vi "Watch_Directory3.vi"() -> ()   [LabVIEW 2015]
uses:
  <vilib>/Utility/config.llb/Read Key (String).vi
  <userlib>/caLab/Private/Get_PV-1D.vi
  <vilib>/Utility/config.llb/NI_LVConfig.lvlib
panel:
  out "Numeric":i32
  out "path":path
  out "concatenated string 8":string
  out "LOGBOOK":string
  out "PATH HSnapjpeg":string
  out "PATH SESdata":string
  out "PV name array":string[](array[string])
  out "BL132:CONFIG":path=path "S:/INI/BL132.INI"
  out "ELOGD_SERVER":string
  out "concatenated string 7":string
  in  "error out 2":errorcluster
  out "error out":errorcluster
  out "EPICS_PVs":string
  out "subarray 2":dbl[](array[numeric])
  out "subarray":dbl[](array[numeric])
  out "concatenated string 3":string
  out "standard error 5":string
  out "standard output 5":string
  out "SEStxt Previous":string
  out "SEStxt":bool
  out "standard output 4":string
  out "standard error 4":string
  out "concatenated string 2":string
  in  "SES_Filter txt":string="*.txt"
  out "SEStxt Current":string
  out "concatenated string 6":string
  out "standard error 3":string
  out "standard output 3":string
  in  "Submit":bool
  in  "HSnap_Filter jpg":string="*.jpg"
  in  "ELOG:HSnap_Maindir":string="S:\\HyperSnap\\"
  out "HSnap Current":string
  out "concatenated string 5":string
  in  "ELOGHSnap_Subdir":string
  out "HSnap Previous":string
  out "HyperSnap":bool
  out "standard output 2":string
  out "standard error 2":string
  out "concatenated string 4":string
  in  "ELOG:SES_maindir":string="P:\\b_ogasawara\\bl13-0\\bl13-2\\dt_SES100\\"
  in  "stop 2":bool
  in  "ELOG_MESSAGE":string caption="Message to ELOG  BL132:Message"
  out "SESpath":path
  in  "ELOG:SES_subdir":string="2017\\BL132\\"
  out "PV Names (dup)":string[](array[string])
  out "concatenated string":string
  out "standard error":string
  out "standard output":string
  out "SESibw":bool
  out "SESibw Previous":string
  in  "SES_Filter ibw":string="*.ibw"
  out "SESibw Current":string
  # "Set a folder to watch using the\nPath control. You can also\nset a filter for a certain type\nof file to watch for (such as\n*.bmp). Then run the\nexample. Whenever you create\na new file in that directory that\nmatches the filter, New File Name\nwill update to let you know the\nnew file name."
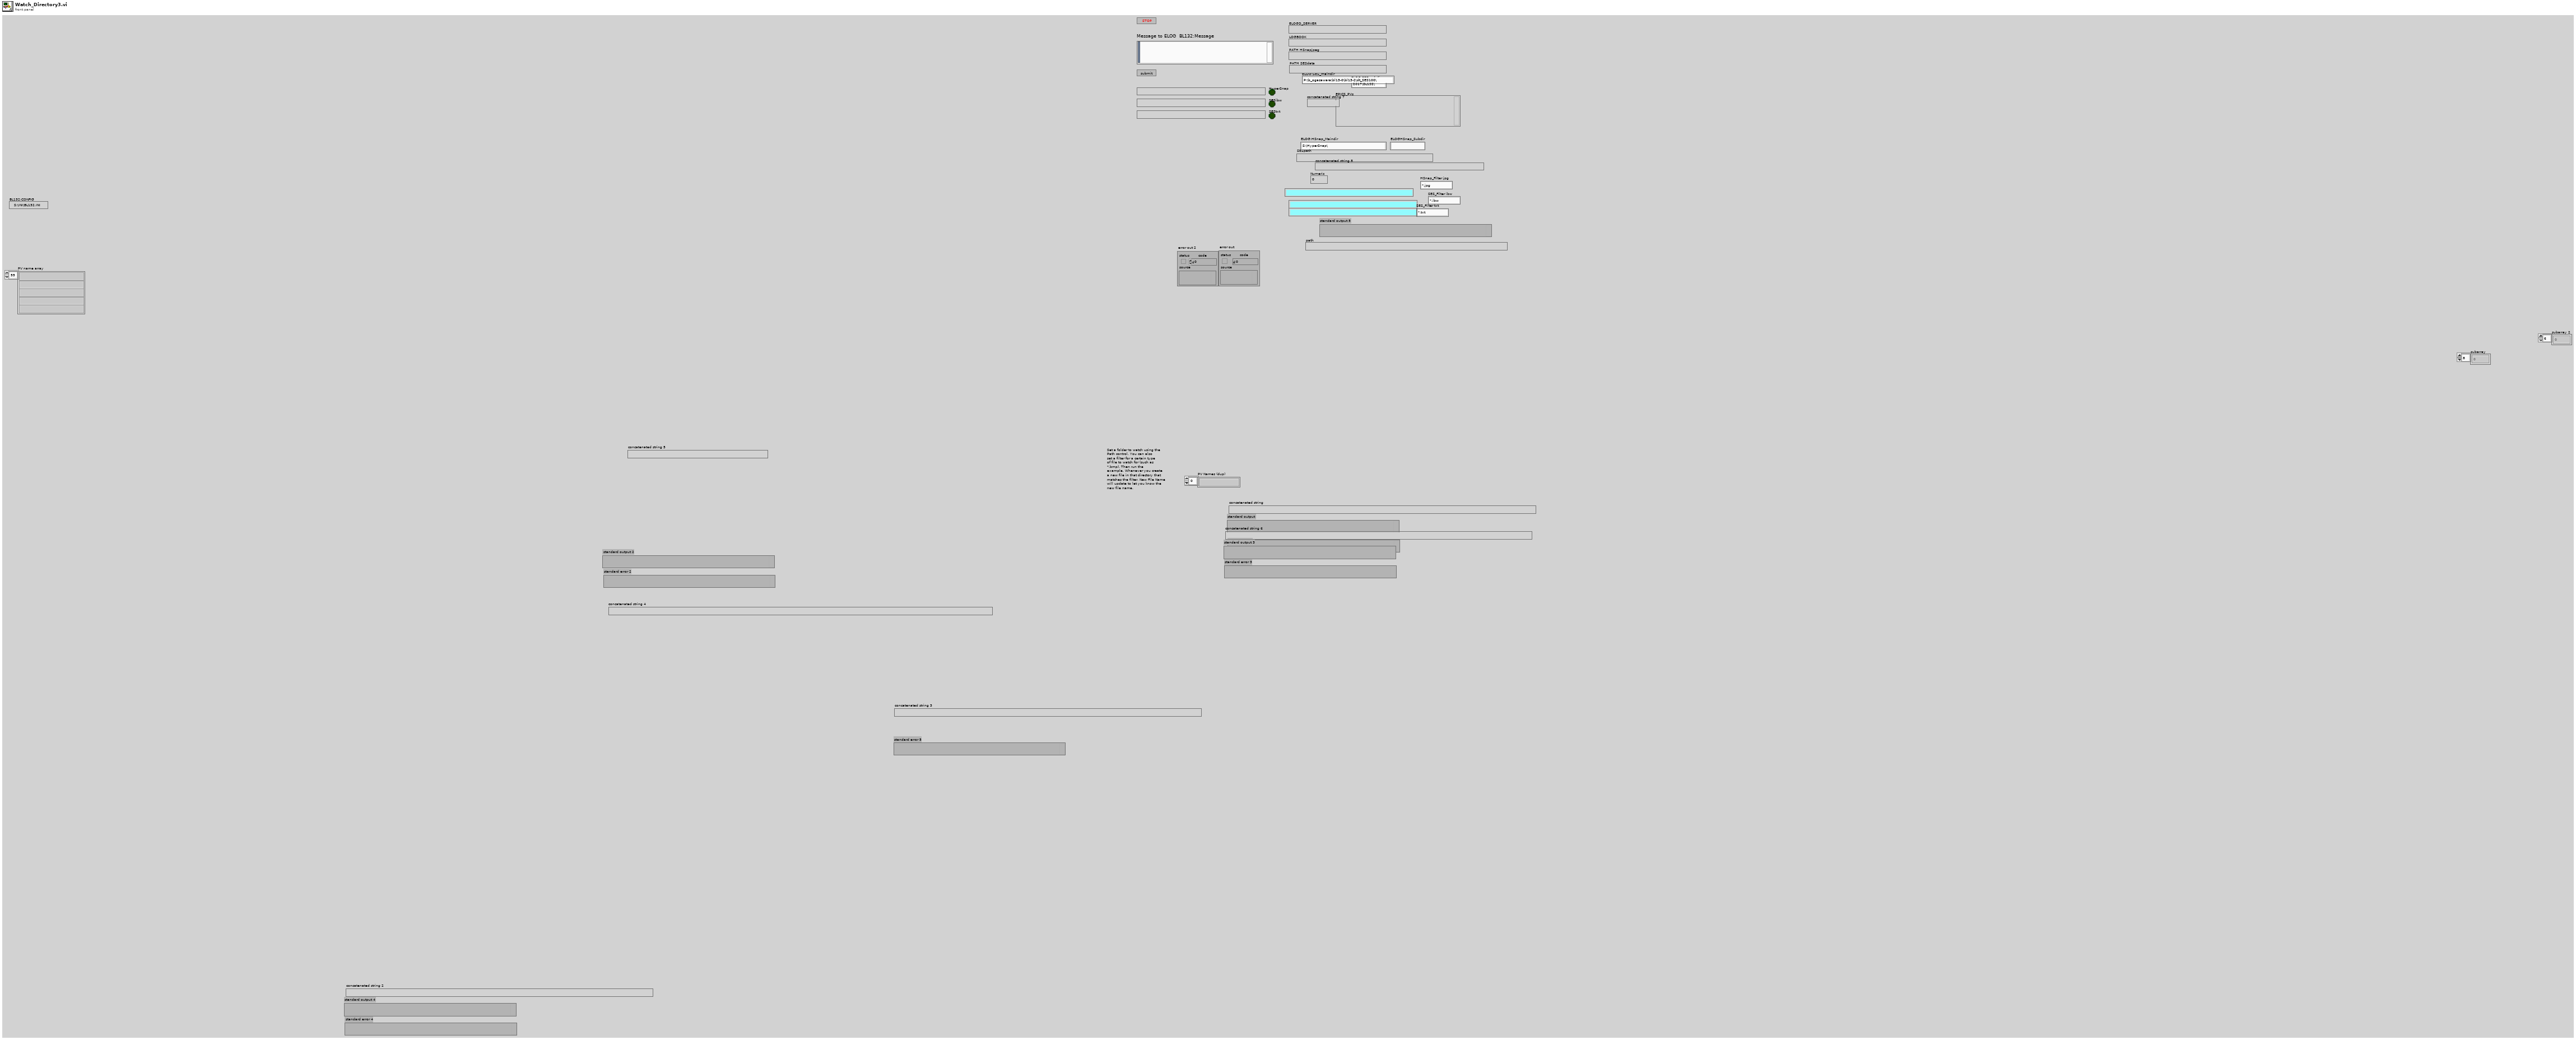
[diagram p1: front panel]
types:
  T1 = typedef "NI_LVConfig.lvlib/Config Data RefNum.ctl" = refnum<k1>
  T2 = enum16{"open", "replace", "create", "open or create", "replace or create", "replace or create with confirmation"}
  T3 = typedef "imagedata.ctl" = cluster{"image type":i32, "image depth":i32, "image":u8[], "mask":u8[], "colors":u32[], "Rectangle":cluster{"left":i16, "top":i16, "right":i16, "bottom":i16}}
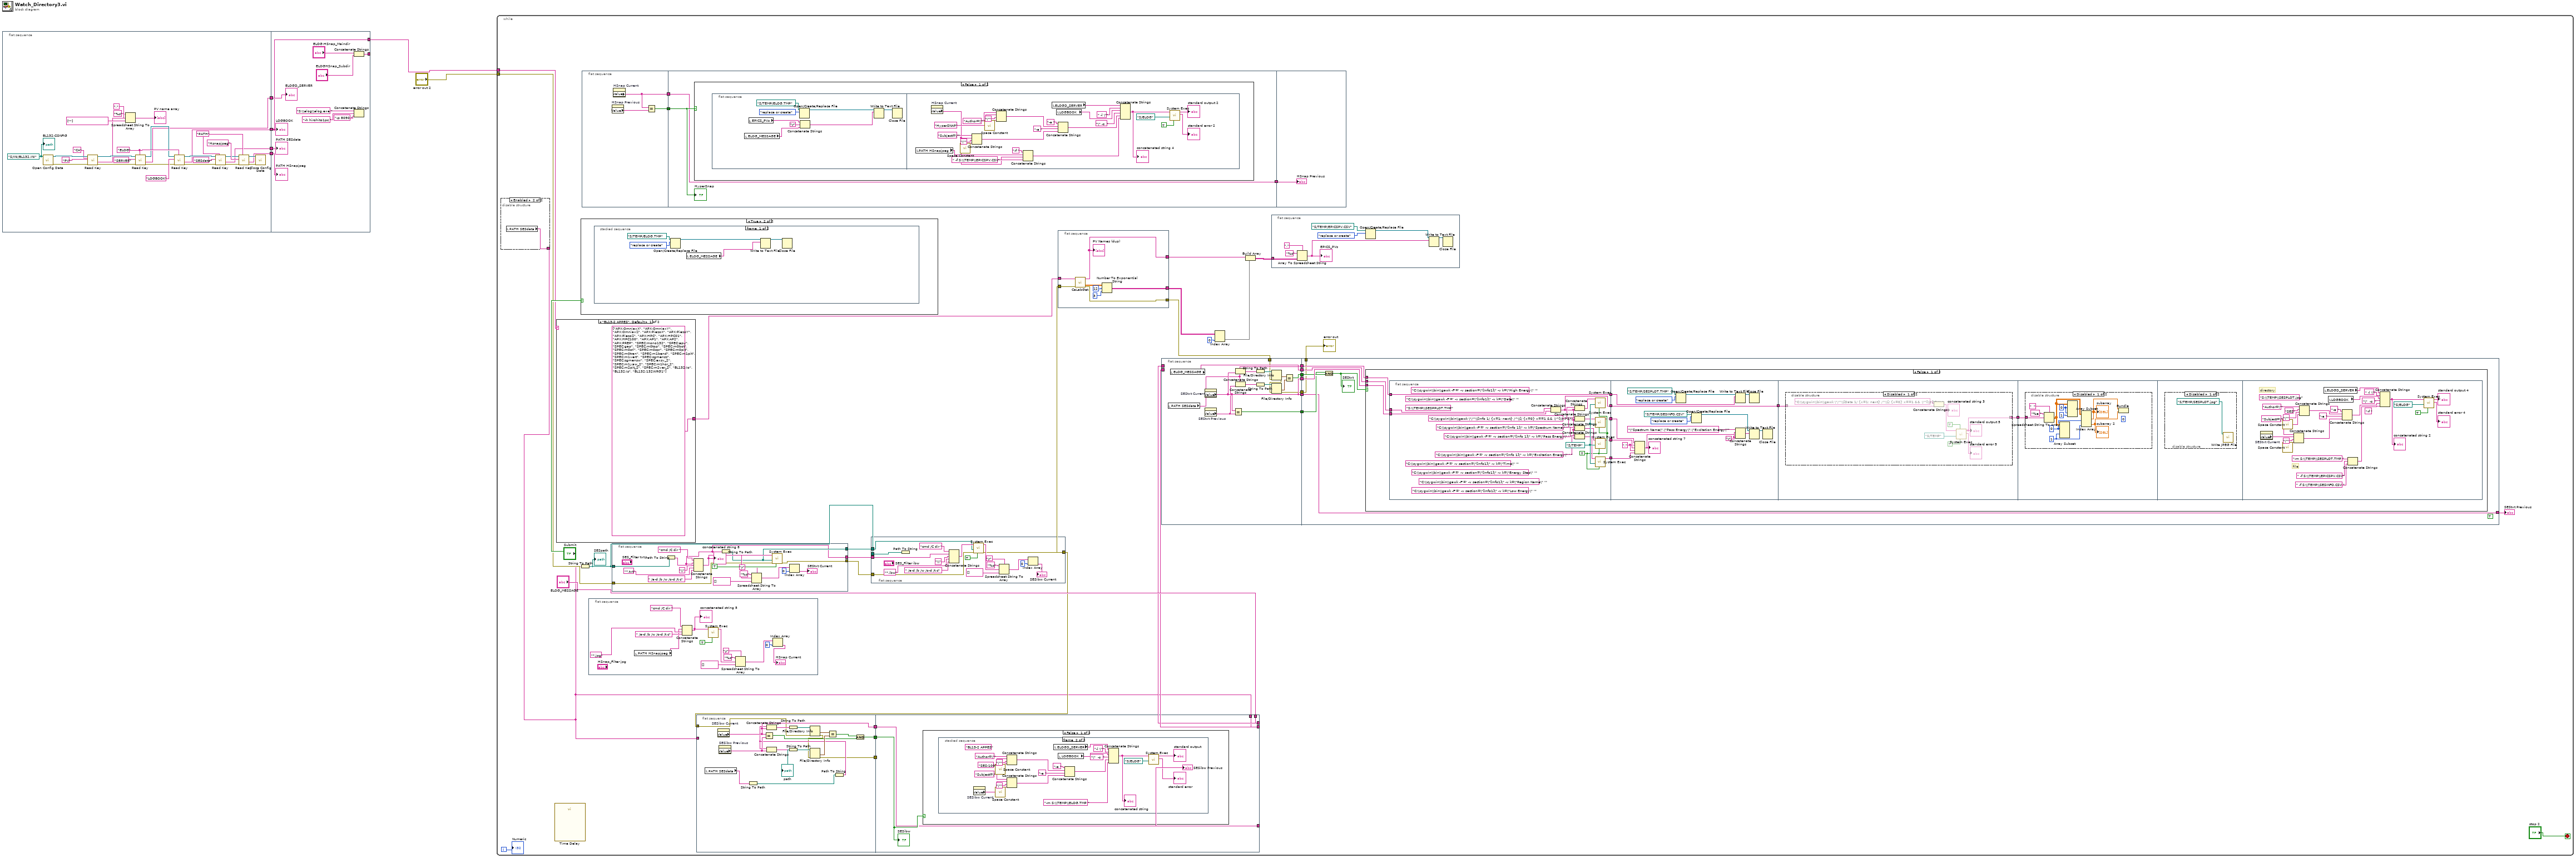
[diagram p0: block diagram]
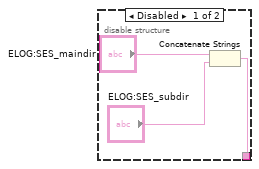
[diagram p2: hidden frame]
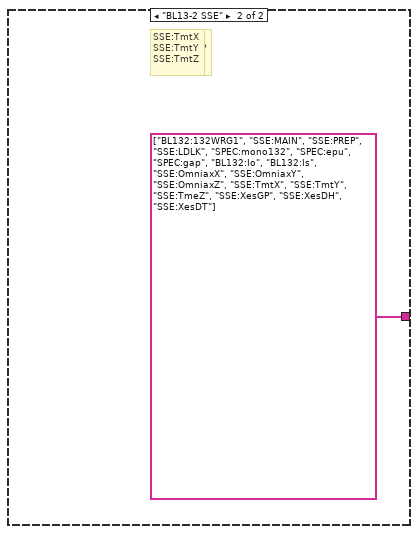
[diagram p3: hidden frame]
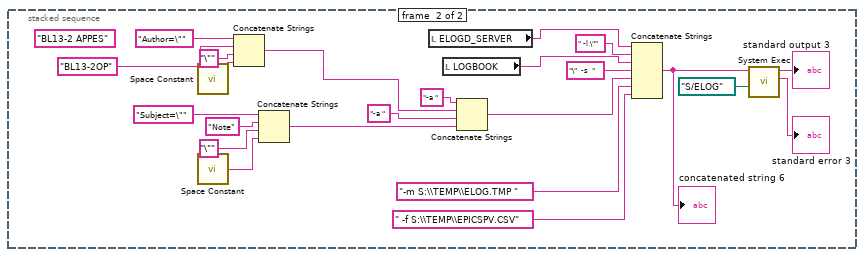
[diagram p9: hidden frame]
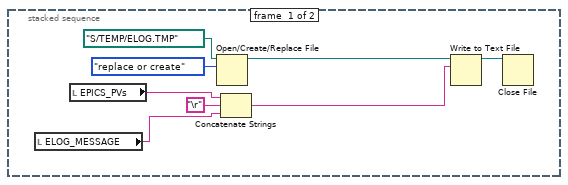
[diagram p11: hidden frame]
diagram:
  n1 = flat-sequence {
    tunnel: [w11] -> w4
    tunnel: [w10] -> w3
    tunnel: [w9] -> w2
    tunnel: [w8] -> w1
    tunnel: [w37] -> w5
    tunnel: [w43] -> _
    tunnel: w4 -> [w40]
    tunnel: w3 -> [w39]
    tunnel: w2 -> [w38]
    tunnel: w1 -> [w37]
    frame #0 {
      w12 = "PATH" ("section")
      w36 = path "S:/INI/BL132.INI" ("configuration file path")
      w18 = "ELOG" ("key")
      n2 = call <vilib>:"Open Config Data.vi"("configuration file path"=w36) -> ("error out"=w25:errorcluster, "refnum"=w33:T1)  [unwired: 8 in, 1 out]
      n3 = call-poly <vilib>:"Read Key.vi"("section"="CA", "error in (no error)"=w25, "key"="PV", "refnum"=w33) -> ("error out"=w26:errorcluster, "value"=w27:string, "refnum out"=w30:T1)  [unwired: 4 in, 1 out]
      n4 = Spreadsheet String To Array(delimiter (Tab)=",", format string="%s", spreadsheet string=w27, array type (2D Dbl)=string[] [""] ("Strings []")) -> (array=→"PV name array":string[])
      n5 = call-poly <vilib>:"Read Key.vi"("section"=w18, "error in (no error)"=w26, "key"="SERVER" ("section"), "refnum"=w30) -> ("error out"=w14:errorcluster, "value"=w9:string, "refnum out"=w16:T1)  [unwired: 4 in, 1 out]
      n6 = call-poly <vilib>:"Read Key.vi"("section"=w18, "error in (no error)"=w14, "key"="LOGBOOK", "refnum"=w16) -> ("error out"=w13:errorcluster, "value"=w8:string, "refnum out"=w15:T1)  [unwired: 4 in, 1 out]
      n7 = call-poly <vilib>:"Read Key.vi"("section"=w12, "error in (no error)"=w13, "key"="SESdata", "refnum"=w15) -> ("error out"=w20:errorcluster, "value"=w11:string, "refnum out"=w22:T1)  [unwired: 4 in, 1 out]
      n8 = call-poly <vilib>:"Read Key.vi"("section"=w12, "error in (no error)"=w20, "key"="Hsnapjpeg", "refnum"=w22) -> ("error out"=w19:errorcluster, "value"=w10:string, "refnum out"=w21:T1)  [unwired: 4 in, 1 out]
      n9 = call <vilib>:"Close Config Data.vi"("error in (no error)"=w19, "refnum"=w21) -> ()  [unwired: 8 in, 2 out]
      "BL132:CONFIG" <- w36
    }
    frame #1 {
      n10 = Concatenate Strings("ELOG:HSnap_Maindir", "ELOGHSnap_Subdir") -> (w43:string)
      n11 = Concatenate Strings("S:\\elog\\elog.exe " ("command line"), "-h hirohito1pc " ("command line"), "-p 8090 " ("string")) -> ()  [unwired: 1 out]
      "ELOGD_SERVER" <- w38
      "PATH SESdata" <- w40
      "PATH HSnapjpeg" <- w39
      "LOGBOOK" <- w37
    }
  }
  n12 = while {
    tunnel: "error out 2" -> [w59]
    tunnel: w5 -> [w56]
    i -> [w47]
    stop <- "stop 2" stop-if-true
    n13 = disable-structure shown="Enabled" {
      disable-tunnel: [w84 w87] -> w48
      frame Disabled {
        n14 = Concatenate Strings("ELOG:SES_maindir", "ELOG:SES_subdir") -> (w84:string)
      }
      frame Enabled {
        n15 = local read "PATH SESdata"() -> (w87:string)
      }
    }
    n16 = call "Time Delay"() -> ()  [unwired: 11 in, 1 out]
    n17 = case shown="\"BL13-2 APPES\", Default" w56 {
      tunnel: [string[] ["APX:OmniaxX", "APX:OmniaxY", "APX:OmniaxZ", "APX:PiezoX", "APX:PiezoY", "APX:PiezoZ", "APX:HPC", "APX:HPC01", "APX:HPC100", "APX:AP1", "APX:AP2", "APX:PREP", "SPEC:mono132", "SPEC:epu", "SPEC:gap", "SPEC:m0top", "SPEC:m0bot", "SPEC:m0srl", "SPEC:m0spr", "SPEC:m0pit", "SPEC:m0tran", "SPEC:m1bend", "SPEC:m1pit", "SPEC:m1vert", "SPEC:sgmensz", "SPEC:sgmensw", "SPEC:exsv_2", "SPEC:m1yaw_2", "SPEC:m1hor_2", "SPEC:m2pit_2", "SPEC:m2ver_2", "BL132:Io", "BL132:Is", "BL132:132WRG1"] string[] ["BL132:132WRG1", "SSE:MAIN", "SSE:PREP", "SSE:LDLK", "SPEC:mono132", "SPEC:epu", "SPEC:gap", "BL132:Io", "BL132:Is", "SSE:OmniaxX", "SSE:OmniaxY", "SSE:OmniaxZ", "SSE:TmtX", "SSE:TmtY", "SSE:TmeZ", "SSE:XesGP", "SSE:XesDH", "SSE:XesDT"]] -> w62
      frame "BL13-2 APPES", Default {
      }
      frame "BL13-2 SSE" {
        # "SSE:TmtX\nSSE:TmtY\nSSE:TmtZ"
        # "SSE:XesDT\nSSE:Xes:GP\nSSE:XesDT"
      }
    }
    n18 = String To Path(string=w48) -> (path=w73:path)
    "SESpath" <- w73
    n19 = case shown="True" "Submit" {
      frame False {
      }
      frame True {
        n20 = stacked-sequence {
          frame #0 {
            n21 = Open/Create/Replace File(file path (use dialog)=path "S:/TEMP/ELOG.TMP", operation (0:open)=T2."replace or create") -> (refnum out=w246:refnum<file>)  [unwired: 4 in, 2 out]
            n22 = local read "ELOG_MESSAGE"() -> (w242:string)
            n23 = Write to Text File(file (use dialog)=w246, text=w242) -> (refnum out=w245:refnum<file>)  [unwired: 2 in, 2 out]
            n24 = Close File(refnum=w245) -> ()  [unwired: 1 in, 2 out]
          }
          frame #1 {
            (unwired) "BL13-2 APPES"
            n25 = call <vilib>:"Space Constant.vi"() -> ("String"=w257:string)
            n26 = call <vilib>:"Space Constant.vi"() -> ("String"=w258:string)
            n27 = Concatenate Strings("Author=\"" ("string"), "BL13-2OP", "\"" ("string"), w257) -> (w255:string)
            n28 = Concatenate Strings("Subject=\"" ("string"), "Note" ("string"), "\"" ("string"), w258) -> (w253:string)
            n29 = local read "ELOGD_SERVER"() -> (w248:string)
            n30 = local read "LOGBOOK"() -> (w247:string)
            n31 = Concatenate Strings("-a ", w255, "-a " ("string"), w253) -> (w254:string)
            n32 = Concatenate Strings(w248, " -l \"" ("command line"), w247, "\"  -s  " ("command line"), w254, "-m S:\\TEMP\\ELOG.TMP " ("string"), " -f S:\\TEMP\\EPICSPV.CSV" ("string")) -> (w266:string)
            "concatenated string 6" <- w266
            n33 = call <vilib>:"System Exec.vi"("working directory"=path "S:/ELOG", "command line"=w266) -> ("standard error"=→"standard error 3":string, "standard output"=→"standard output 3":string)  [unwired: 6 in, 2 out]
          }
        }
      }
    }
    n34 = flat-sequence {
      tunnel: [w283] -> w81
      tunnel: [w284] -> w80
      tunnel: w81 -> [w286]
      tunnel: [w286] -> w79
      tunnel: w80 -> [w287]
      tunnel: w79 -> [w322]
      frame #0 {
        n35 = property on="HSnap Previous" class="Str"() -> ("Value"=w285:string)  [unwired: 2 in, 2 out]
        n36 = property on="HSnap Current" class="Str"() -> ("Value"=w283:string)  [unwired: 2 in, 2 out]
        n37 = Equal?(x=w283, y=w285) -> (x = y?=w284:bool)
      }
      frame #1 {
        n38 = case shown="False" w287 {
          frame False {
            n39 = flat-sequence {
              frame #0 {
                n40 = local read "ELOG_MESSAGE"() -> (w288:string)
                n41 = local read "EPICS_PVs"() -> (w289:string)
                n42 = Open/Create/Replace File(file path (use dialog)=path "S:/TEMP/ELOG.TMP", operation (0:open)=T2."replace or create") -> (refnum out=w295:refnum<file>)  [unwired: 4 in, 2 out]
                n43 = Concatenate Strings(w289, "\r", w288) -> (w290:string)
                n44 = Write to Text File(file (use dialog)=w295, text=w290) -> (refnum out=w294:refnum<file>)  [unwired: 2 in, 2 out]
                n45 = Close File(refnum=w294) -> ()  [unwired: 1 in, 2 out]
              }
              frame #1 {
                n46 = local read "PATH HSnapjpeg"() -> (w297:string)
                n47 = property on="HSnap Current" class="Str"() -> ("Value"=w296:string)  [unwired: 2 in, 2 out]
                n48 = call <vilib>:"Space Constant.vi"() -> ("String"=w304:string)
                n49 = Concatenate Strings("Subject=\"" ("string"), w296, "\"" ("string"), w304) -> (w306:string)
                n50 = call <vilib>:"Space Constant.vi"() -> ("String"=w310:string)
                n51 = Concatenate Strings("Author=\"" ("string"), "HyperSNAP", "\"" ("string"), w310) -> (w308:string)
                n52 = Concatenate Strings("-f " ("string"), w297, w296, " -f S:\\TEMP\\EPICSPV.CSV" ("string")) -> (w299:string)
                n53 = local read "ELOGD_SERVER"() -> (w298:string)
                n54 = local read "LOGBOOK"() -> (w302:string)
                n55 = Concatenate Strings("-a ", w308, "-a " ("string"), w306) -> (w307:string)
                n56 = Concatenate Strings(w298, " -l \"" ("command line"), w302, "\" -s  " ("command line"), w307, w299) -> (w318:string)
                "concatenated string 4" <- w318
                n57 = call <vilib>:"System Exec.vi"("run minimized? (F)"=TRUE, "working directory"=path "S:/ELOG", "command line"=w318) -> ("standard error"=→"standard error 2":string, "standard output"=→"standard output 2":string)  [unwired: 5 in, 2 out]
              }
            }
          }
          frame True {
          }
        }
        "HyperSnap" <- w287
      }
      frame #2 {
        "HSnap Previous" <- w322
      }
    }
    n58 = flat-sequence {
      frame #0 {
        n59 = local read "PATH HSnapjpeg"() -> (w270:string)
        n60 = Concatenate Strings("cmd /C dir " ("command line"), w270, "*.jpg" ("HSnap_Filter jpg"), " /a-d /b /w /o-d /t c" ("command line")) -> (w277:string)
        "concatenated string 5" <- w277
        n61 = call <vilib>:"System Exec.vi"("run minimized? (F)"=TRUE, "command line"=w277) -> ("standard output"=w281:string)  [unwired: 4 in, 5 out]
        n62 = Spreadsheet String To Array(delimiter (Tab)="\r", format string="%s", spreadsheet string=w281, array type (2D Dbl)=string[] []) -> (array=w276:string[])
        n63 = Index Array(array=w276, index=0) -> (element=→"HSnap Current":string)
      }
    }
    n64 = flat-sequence {
      tunnel: w73 -> [w235]
      tunnel: w59 -> [w231]
      tunnel: [w230] -> w57
      tunnel: [w227] -> w55
      tunnel: [w224] -> w53
      frame #0 {
        n65 = Path To String(path=w235) -> (string=w224:string)
        n66 = Concatenate Strings("cmd /C dir " ("command line"), w224, "\\" ("string"), "*.txt" ("HSnap_Filter jpg"), " /a-d /b /w /o-d /t c" ("command line")) -> (w236:string)
        "concatenated string 8" <- w236
        n67 = String To Path(string=w224) -> (path=w227:path)
        n68 = call <vilib>:"System Exec.vi"("run minimized? (F)"=TRUE, "error in (no error)"=w231, "working directory"=w227, "command line"=w236) -> ("error out"=w230:errorcluster, "standard output"=w240:string)  [unwired: 2 in, 4 out]
        n69 = Spreadsheet String To Array(delimiter (Tab)="\r", format string="%s", spreadsheet string=w240, array type (2D Dbl)=string[] []) -> (array=w234:string[])
        n70 = Index Array(array=w234, index=0) -> (element=→"SEStxt Current":string)
      }
    }
    n71 = flat-sequence {
      tunnel: [w351] -> w83
      tunnel: w48 -> [_]
      tunnel: [w347] -> w63
      tunnel: w54 -> [w343]
      tunnel: [w341] -> w52
      tunnel: [w361] -> w66
      tunnel: w48 -> [w361]
      tunnel: [w360] -> w65
      tunnel: "ELOG_MESSAGE" -> [w360]
      tunnel: w83 -> [w358]
      tunnel: w63 -> [w359]
      tunnel: [w358] -> w61
      tunnel: w52 -> [_]
      frame #0 {
        n72 = local read "PATH SESdata"() -> (w346:string)
        n73 = property on="SESibw Current" class="Str"() -> ("Value"=w351:string)  [unwired: 2 in, 2 out]
        n74 = property on="SESibw Previous" class="Str"() -> ("Value"=w350:string)  [unwired: 2 in, 2 out]
        n75 = String To Path(string=w346) -> (path=w345:path)
        n76 = Equal?(x=w351, y=w350) -> (x = y?=w348:bool)
        n77 = Path To String(path=w345) -> (string=w344:string)
        n78 = Concatenate Strings(w344, w351) -> (w354:string)
        n79 = Concatenate Strings(w344, w350) -> (w355:string)
        n80 = String To Path(string=w354) -> (path=w357:path)
        n81 = String To Path(string=w355) -> (path=w356:path)
        "path" <- w356
        n82 = File/Directory Info(path=w357, error in=w343) -> (last mod=w353:timestamp, error out=w342:errorcluster)  [unwired: 5 out]
        n83 = File/Directory Info(path=w356, error in=w342) -> (last mod=w352:timestamp, error out=w341:errorcluster)  [unwired: 5 out]
        n84 = Equal?(x=w353, y=w352) -> (x = y?=w349:bool)
        n85 = And(x=w349, y=w348) -> (x .and. y?=w347:bool)
      }
      frame #1 {
        n86 = case shown="False" w359 {
          frame False {
            n87 = stacked-sequence {
              frame #0 {
                n88 = local read "ELOG_MESSAGE"() -> (w362:string)
                n89 = local read "EPICS_PVs"() -> (w363:string)
                n90 = Open/Create/Replace File(file path (use dialog)=path "S:/TEMP/ELOG.TMP", operation (0:open)=T2."replace or create") -> (refnum out=w369:refnum<file>)  [unwired: 4 in, 2 out]
                n91 = Concatenate Strings(w363, "\r", w362) -> (w364:string)
                n92 = Write to Text File(file (use dialog)=w369, text=w364) -> (refnum out=w368:refnum<file>)  [unwired: 2 in, 2 out]
                n93 = Close File(refnum=w368) -> ()  [unwired: 1 in, 2 out]
              }
              frame #1 {
                (unwired) "BL13-2 APPES"
                n94 = property on="SESibw Current" class="Str"() -> ("Value"=w373:string)  [unwired: 2 in, 2 out]
                n95 = call <vilib>:"Space Constant.vi"() -> ("String"=w379:string)
                n96 = call <vilib>:"Space Constant.vi"() -> ("String"=w380:string)
                n97 = Concatenate Strings("Author=\"" ("string"), "SES-100", "\"" ("string"), w379) -> (w377:string)
                n98 = Concatenate Strings("Subject=\"" ("string"), w373, "\"" ("string"), w380) -> (w375:string)
                n99 = local read "ELOGD_SERVER"() -> (w371:string)
                n100 = local read "LOGBOOK"() -> (w370:string)
                n101 = Concatenate Strings("-a ", w377, "-a " ("string"), w375) -> (w376:string)
                n102 = Concatenate Strings(w371, "-l \"" ("command line"), w370, "\"  -s  " ("command line"), w376, "-m S:\\TEMP\\ELOG.TMP " ("string")) -> (w388:string)
                "concatenated string" <- w388
                n103 = call <vilib>:"System Exec.vi"("working directory"=path "S:/ELOG", "command line"=w388) -> ("standard error"=→"standard error":string, "standard output"=→"standard output":string)  [unwired: 6 in, 2 out]
              }
            }
          }
          frame True {
          }
        }
        "SESibw" <- w359
      }
    }
    n104 = flat-sequence {
      tunnel: w73 -> [w334]
      tunnel: w57 -> [w330]
      tunnel: [w329] -> w54
      tunnel: w55 -> [w326]
      tunnel: w53 -> [w323]
      frame #0 {
        n105 = Path To String(path=w334) -> ()  [unwired: 1 out]
        n106 = Concatenate Strings("cmd /C dir " ("command line"), w323, "\\" ("string"), "*.ibw" ("SES_Filter ibw"), " /a-d /b /w /o-d /t c" ("command line")) -> (w335:string)
        n107 = call <vilib>:"System Exec.vi"("run minimized? (F)"=TRUE, "error in (no error)"=w330, "working directory"=w326, "command line"=w335) -> ("error out"=w329:errorcluster, "standard output"=w339:string)  [unwired: 2 in, 4 out]
        n108 = Spreadsheet String To Array(delimiter (Tab)="\r", format string="%s", spreadsheet string=w339, array type (2D Dbl)=string[] []) -> (array=w333:string[])
        n109 = Index Array(array=w333, index=0) -> (element=→"SESibw Current":string)
      }
    }
    n110 = flat-sequence {
      tunnel: [w103] -> w77
      tunnel: [w102] -> w75
      tunnel: w62 -> [w101]
      tunnel: w54 -> [w99]
      tunnel: [w98] -> w50
      frame #0 {
        n111 = call-poly <userlib>:"CaLabGet.vi"("PV Names"=w101, "Error in (no error)"=w99) -> ("PV Names (dup)"=w102:string[], "Value Array (number)"=w100:dbl[][], "Error out"=w98:errorcluster)  [unwired: 7 in, 4 out]
        "PV Names (dup)" <- w102
        n112 = Number To Exponential String(number=w100, precision (6)=i16 3, 3:i16 12 ("width (-)")) -> (E-format string=w103:string[][])  [unwired: 1 in]
      }
    }
    n113 = flat-sequence {
      tunnel: [w117] -> w72
      tunnel: [w120] -> w71
      tunnel: [w110] -> w70
      tunnel: [w117] -> w69
      tunnel: [w109] -> w68
      tunnel: w66 -> [_]
      tunnel: w65 -> [_]
      tunnel: [w111] -> w64
      tunnel: [w107] -> w51
      tunnel: w50 -> [w106]
      tunnel: w72 -> [w122]
      tunnel: w71 -> [w124]
      tunnel: w70 -> [w128]
      tunnel: w69 -> [w127]
      tunnel: w68 -> [w126]
      tunnel: w64 -> [w125]
      tunnel: [w122] -> w60
      tunnel: w51 -> [w121]
      tunnel: [w121] -> w49
      frame #0 {
        n114 = local read "PATH SESdata"() -> (w110:string)
        n115 = local read "ELOG_MESSAGE"() -> (w109:string)
        n116 = property on="SEStxt Current" class="Str"() -> ("Value"=w117:string)  [unwired: 2 in, 2 out]
        n117 = property on="SEStxt Previous" class="Str"() -> ("Value"=w116:string)  [unwired: 2 in, 2 out]
        n118 = Equal?(x=w117, y=w116) -> (x = y?=w120:bool)
        n119 = Concatenate Strings(w110, w117) -> (w114:string)
        n120 = Concatenate Strings(w110, w116) -> (w115:string)
        n121 = String To Path(string=w114) -> (path=w119:path)
        n122 = String To Path(string=w115) -> (path=w118:path)
        n123 = File/Directory Info(path=w119, error in=w106) -> (last mod=w113:timestamp, error out=w108:errorcluster)  [unwired: 5 out]
        n124 = File/Directory Info(path=w118, error in=w108) -> (last mod=w112:timestamp, error out=w107:errorcluster)  [unwired: 5 out]
        n125 = Equal?(x=w113, y=w112) -> (x = y?=w111:bool)
      }
      frame #1 {
        (unwired) TRUE
        n126 = And(x=w124, y=w125) -> (x .and. y?=w123:bool)
        "SEStxt" <- w123
        n127 = case shown="False" w123 {
          tunnel: w126 -> [w138 _]
          tunnel: w128 -> [w137 _]
          tunnel: w127 -> [w136 _]
          frame False {
            n128 = flat-sequence {
              tunnel: w138 -> [w151]
              tunnel: w137 -> [w153]
              tunnel: w136 -> [w152]
              tunnel: [w147] -> w134
              tunnel: [w151] -> w132
              tunnel: [w141] -> w131
              tunnel: [w140] -> w130
              tunnel: [w139] -> w129
              tunnel: w134 -> [w173]
              tunnel: [w173] -> w133
              tunnel: w132 -> [w166]
              tunnel: w131 -> [w165]
              tunnel: w130 -> [w164]
              tunnel: w129 -> [w163]
              tunnel: w133 -> [w175]
              tunnel: [w174] -> w135
              tunnel: w135 -> [w184]
              frame #0 {
                (unwired) "C:\\cygwin\\bin\\gawk -F'=' -v section=\"[Info1]\" -v k=\"Energy Step\" '" ("command line")
                (unwired) "C:\\cygwin\\bin\\gawk -F'=' -v section=\"[Info1]\" -v k=\"Low Energy\" '" ("command line")
                (unwired) "C:\\cygwin\\bin\\gawk -F'=' -v section=\"[Info1]\" -v k=\"High Energy\" '" ("command line")
                (unwired) "C:\\cygwin\\bin\\gawk -F'=' -v section=\"[Info1]\" -v k=\"Time\" '" ("command line")
                (unwired) "C:\\cygwin\\bin\\gawk -F'=' -v section=\"[Info1]\" -v k=\"Date\" '" ("command line")
                (unwired) "C:\\cygwin\\bin\\gawk -F'=' -v section=\"[Info1]\" -v k=\"Region Name\" '" ("command line")
                w142 = TRUE ("run minimized? (F)")
                (unwired) "S:\\TEMP\\SESPPLOT.TMP" ("string")
                w146 = path "S:/TEMP" ("working directory")
                n129 = Concatenate Strings(w153, w152) -> (w147:string)
                n130 = Concatenate Strings("C:\\cygwin\\bin\\gawk \"/^\\[Info 1/ {x=1; next} /^\\[/ {x=0} x==1 && !/^[\\t ]*$/\" " ("command line"), w147) -> (w154:string)
                n131 = Concatenate Strings("C:\\cygwin\\bin\\gawk -F'=' -v section=\"[Info 1]\" -v k=\"Spectrum Name\" ' " ("command line"), w147) -> (w145:string)
                n132 = Concatenate Strings("C:\\cygwin\\bin\\gawk -F'=' -v section=\"[Info 1]\" -v k=\"Pass Energy\" ' " ("command line"), w147) -> (w144:string)
                n133 = Concatenate Strings("C:\\cygwin\\bin\\gawk -F'=' -v section=\"[Info 1]\" -v k=\"Excitation Energy\" ' " ("command line"), w147) -> (w143:string)
                n134 = call <vilib>:"System Exec.vi"("run minimized? (F)"=w142, "working directory"=w146, "command line"=w154) -> ()  [unwired: 5 in, 4 out]
                n135 = call <vilib>:"System Exec.vi"("run minimized? (F)"=w142, "working directory"=w146, "command line"=w145) -> ("standard output"=w141:string)  [unwired: 5 in, 3 out]
                n136 = call <vilib>:"System Exec.vi"("run minimized? (F)"=w142, "working directory"=w146, "command line"=w144) -> ("standard output"=w140:string)  [unwired: 5 in, 3 out]
                n137 = call <vilib>:"System Exec.vi"("run minimized? (F)"=w142, "working directory"=w146, "command line"=w143) -> ("standard output"=w139:string)  [unwired: 5 in, 3 out]
              }
              frame #1 {
                w162 = "," ("string")
                w171 = "\r"
                n138 = Concatenate Strings(w165, w162, w164, w162, w163) -> (w161:string)
                "concatenated string 7" <- w161
                n139 = Open/Create/Replace File(file path (use dialog)=path "S:/TEMP/SESPLOT.TMP", operation (0:open)=T2."replace or create") -> (refnum out=w172:refnum<file>)  [unwired: 4 in, 2 out]
                n140 = Open/Create/Replace File(file path (use dialog)=path "S:/TEMP/SESINFO.CSV", operation (0:open)=T2."replace or create") -> (refnum out=w157:refnum<file>)  [unwired: 4 in, 2 out]
                n141 = Write to Text File(file (use dialog)=w172, text=w166) -> (refnum out=w168:refnum<file>)  [unwired: 2 in, 2 out]
                n142 = Concatenate Strings("\"Spectrum Name\",\"Pass Energy\",\"Excitation Energy\"", w171, w161, w171) -> (w156:string)
                n143 = Close File(refnum=w168) -> ()  [unwired: 1 in, 2 out]
                n144 = Write to Text File(file (use dialog)=w157, text=w156) -> (refnum out=w158:refnum<file>)  [unwired: 2 in, 2 out]
                n145 = Close File(refnum=w158) -> ()  [unwired: 1 in, 2 out]
              }
              frame #2 {
                n146 = disable-structure shown="Disabled" {
                  disable-tunnel: w175 -> [w179 _]
                  disable-tunnel: [w177 _] -> w174
                  frame Disabled {
                    n147 = Concatenate Strings("C:\\cygwin\\bin\\gawk \"/^\\[Data 1/ {x=1; next} /^\\[/ {x=0} x==1 && !/^[\\t ]*$/\" " ("command line"), w179) -> (w183:string)
                    "concatenated string 3" <- w183
                    n148 = call <vilib>:"System Exec.vi"("run minimized? (F)"=TRUE, "wait until completion? (T)"=TRUE, "working directory"=path "S:/TEMP", "command line"=w183) -> ("standard error"=→"standard error 5":string, "standard output"=w177:string)  [unwired: 4 in, 2 out]
                    "standard output 5" <- w177
                  }
                  frame Enabled {
                  }
                }
              }
              frame #3 {
                n149 = disable-structure shown="Disabled" {
                  disable-tunnel: w184 -> [w185 _]
                  frame Disabled {
                    (unwired) 0 ("index")
                    w190 = 1 ("index")
                    w189 = 0 ("index")
                    w193 = 0 ("index")
                    n150 = Spreadsheet String To Array(delimiter (Tab)="  " ("format string"), format string="%e ", spreadsheet string=w185) -> (array=w191:dbl[][])  [unwired: 1 in]
                    n151 = Array Subset(array=w191, index (row)=w189, index (col)=w190) -> ()  [unwired: 2 in, 1 out]
                    n152 = Array Subset(array=w191, index (row)=w193, index (col)=w193, length (col)=1 ("index")) -> ()  [unwired: 1 in, 1 out]
                    n153 = Index Array(array=w191, index (col) #1=w189, index (col) #2=w190) -> (element #1=w188:dbl[], element #2=w187:dbl[])  [unwired: 2 in]
                    "subarray" <- w188
                    "subarray 2" <- w187
                    n154 = Bundle(w188, w187) -> (w186:cluster{dbl[], dbl[]})  [unwired: 1 in]
                  }
                  frame Enabled {
                  }
                }
              }
              frame #4 {
                n155 = disable-structure shown="Disabled" {
                  frame Disabled {
                    n156 = call <vilib>:"Write JPEG File.vi"("path to JPEG file"=path "S:/TEMP/SESPLOT.jpg" ("file path (use dialog)")) -> ("image data"=w196:T3)  [unwired: 8 in, 2 out]
                  }
                  frame Enabled {
                  }
                }
              }
              frame #5 {
                (unwired) "S:\\TEMP\\SESPLOT.jpg" ("string")
                (unwired) "-f " ("string")
                # "file"
                # "directory"
                n157 = property on="SEStxt Current" class="Str"() -> ("Value"=w206:string)  [unwired: 2 in, 2 out]
                n158 = call <vilib>:"Space Constant.vi"() -> ("String"=w212:string)
                n159 = call <vilib>:"Space Constant.vi"() -> ("String"=w213:string)
                n160 = Concatenate Strings("Subject=\"" ("string"), w206, "\"" ("string"), w213) -> (w208:string)
                n161 = Concatenate Strings("Author=\"" ("string"), "SES", "\"" ("string"), w212) -> (w210:string)
                n162 = local read "ELOGD_SERVER"() -> (w198:string)
                n163 = local read "LOGBOOK"() -> (w205:string)
                n164 = Concatenate Strings("-a ", w210, "-a " ("string"), w208) -> (w209:string)
                n165 = Concatenate Strings("-m S:\\TEMP\\SESPLOT.TMP " ("string"), " -f S:\\TEMP\\EPICSPV.CSV" ("string"), " -f S:\\TEMP\\SESINFO.CSV " ("string")) -> (w202:string)
                n166 = Concatenate Strings(w198, " -l \"" ("command line"), w205, "\"  -s  " ("command line"), w209, w202) -> (w221:string)
                "concatenated string 2" <- w221
                n167 = call <vilib>:"System Exec.vi"("run minimized? (F)"=TRUE, "working directory"=path "S:/ELOG", "command line"=w221) -> ("standard error"=→"standard error 4":string, "standard output"=→"standard output 4":string)  [unwired: 5 in, 2 out]
              }
            }
          }
          frame True {
          }
        }
      }
    }
    n168 = Index Array(array=w77, index (col)=0) -> (element=w78:string[])  [unwired: 1 in]
    n169 = Build Array "Build Array"(w75, w78) -> (w58:string[][])
    n170 = flat-sequence {
      tunnel: w58 -> [w88]
      frame #0 {
        n171 = Array To Spreadsheet String(delimiter (Tab)=",", array=w88, 3:"%s" ("format string")) -> (spreadsheet string=w89:string)
        "EPICS_PVs" <- w89
        n172 = Open/Create/Replace File(file path (use dialog)=path "S:/TEMP/EPICSPV.CSV", operation (0:open)=T2."replace or create") -> (refnum out=w90:refnum<file>)  [unwired: 4 in, 2 out]
        n173 = Write to Text File(file (use dialog)=w90, text=w89) -> (refnum out=w91:refnum<file>)  [unwired: 2 in, 2 out]
        n174 = Close File(refnum=w91) -> ()  [unwired: 1 in, 2 out]
      }
    }
    "SESibw Previous" <- w61
    "SEStxt Previous" <- w60
    "error out" <- w49
    "Numeric" <- w47
  }
